vi "Calculate Feedforward.vi"() -> ()   [LabVIEW 2015]
uses:
  <vilib>/Rock Robotics/WPI/CAN/TalonSRX/WPI_CANTalonSRX_APIControlMode.ctl
  <vilib>/Rock Robotics/WPI/MotorControl/WPI_MotorControlOpenCANTalonSRX.vi
panel:
  out "Deltas":dbl[](array[numeric])
  out "Sensor Velocity":dbl[](array[numeric])
  out "Motor Setpoints":dbl[](array[numeric])
  out "Feedfoward(s)":dbl[](array[numeric])
  in  "Motor Inverts":bool[](array[boolean])
  in  "Motor IDs":u8[][](array[numeric])
  out "Valid Data":bool
  out "Velocity Chart (in array order)":cluster{"[0]":dbl, "[1]":dbl}(graph)
  in  "Target Output (vbus)":dbl=0.5 format="%#_13g"
  in  "Counts per rev of encoder":i32=1024
  in  "stop":bool
  in  "Start":bool
  in  "size of averaging array":i32
  in  "Valid Delta":dbl format="%#_13g"
  # "The first of every row is the master motor and every motor after that is the slave to thr"
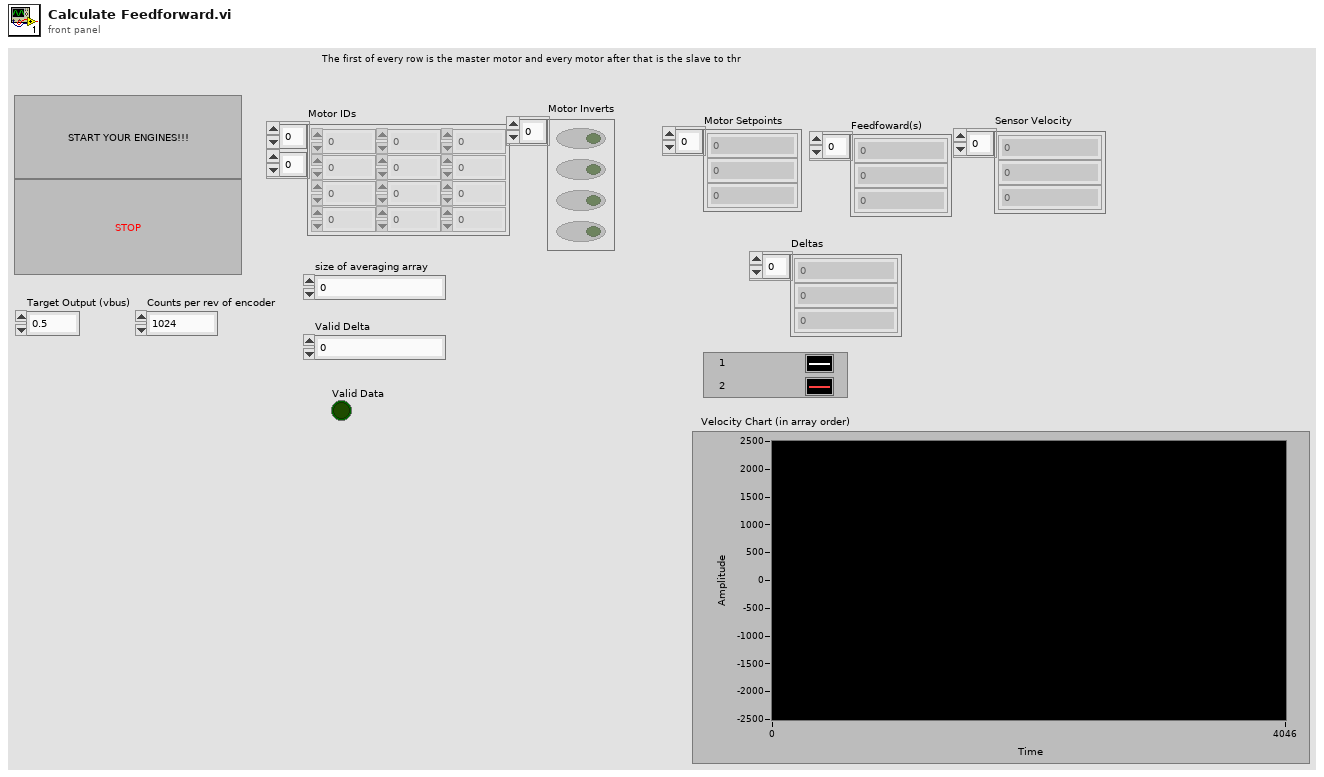
[diagram p1: front panel]
types:
  T1 = typedef "WPI_CANTalonSRX_APIControlMode.ctl" = enum8{"Percent VBus", "Speed", "Position", "Slave", "Unchanged / Invalid", "Voltage Compensation", "Current", "Motion Profile"}
  T2 = typedef "WPI_MotorControlDeviceRef.ctl" = cluster{"DeviceStatus":errorcluster, "Type":T3, "PWM":cluster{"PWM Channel":T4, "DeadBand":T5}, "CAN":cluster{"Device Number":u8, "Control Mode":T6, "Semaphore":T7, "Max Vout":dbl, "TalonSRX Control Mode":T1}, "Invert":bool}
  T3 = typedef "WPI_MotorControlType.ctl" = enum16{"PWM", "CAN", "CANTalonSRX"}
  T4 = typedef "FPGA_DIOPWMChannel.ctl" = enum8{"PWM 0", "PWM 1", "PWM 2", "PWM 3", "PWM 4", "PWM 5", "PWM 6", "PWM 7", "PWM 8", "PWM 9", "PWM MXP 0", "PWM MXP 1", "PWM MXP 2", "PWM MXP 3", "PWM MXP 4", "PWM MXP 5", "PWM MXP 6", "PWM MXP 7", "PWM MXP 8", "PWM MXP 9", "Invalid"}
  T5 = typedef "WPI_PWMDeadband.ctl" = cluster{"Name":string, "maxPositivePwm":i32, "minPositivePwm":i32, "centerPwm":i32, "maxNegativePwm":i32, "minNegativePwm":i32, "angularRange":u16}
  T6 = typedef "WPI_CANJaguar_ControlMode.ctl" = enum8{"Percent VBus", "Current", "Speed", "Position", "Voltage"}
  T7 = typedef "Semaphore RefNum" = refnum<k1>
  T8 = typedef "WPI_CANTalonSRX_GlobalStatus.ctl" = cluster{"Applied Throttle":dbl, "Module Enabled":bool, "CAN Error":errorcluster, "Closed Loop Error":dbl, "Forward Limit Switch Closed":bool, "Reverse Limit Switch Closed":bool, "Sensor Position":dbl, "Sensor Velocity":dbl, "Current":dbl, "Sticky Fault - Over Temp":bool, "Sticky Fault - Under Voltage":bool, "Sticky Fault - Forward Limit":bool, "Sticky Fault - Reverse Limit":bool, "Sticky Fault - Forward Soft Limit":bool, "Sticky Fault - Reverse Soft Limit":bool, "Brake is Enabled":bool, "Encoder Position":dbl, "Encoder Velocity":dbl, "Encoder Index Count":dbl, "Encoder A Pin State":bool, "Encoder B Pin State":bool, "Encoder Index Pin State":bool, "Analog In":dbl, "Analog In Velocity":dbl, "Temperature (C)":dbl, "Battery Voltage":dbl, "Control 5 Is Supported":bool, "Current Profile Slot Select":dbl, "Pos Div 8":bool, "Vel Div 4":bool, "Pulse Width Position":i32, "Pulse Width Velocity":i32, "Pulse Width Rise To Rise (us)":i32, "Pulse Width Rise To Fall (us)":i32, "Mot Prof Active Is Under Run":bool, "Mot Prof Active Has Under Run":bool, "Mot Prof Active Is Last":bool, "Mot Prof Active Velocity Only":bool, "Mot Prof Active Is Valid":bool, "Mot Prof Buffer Is Full":bool, "Mot Prof Active Profile Slot Select":i32, "Mot Prof NextID":i32, "Mot Prof Count":i32, "Mot Prof Active Velocity":dbl, "Mot Prof Active Position":dbl, "Mot Prof Output Enable":i32}
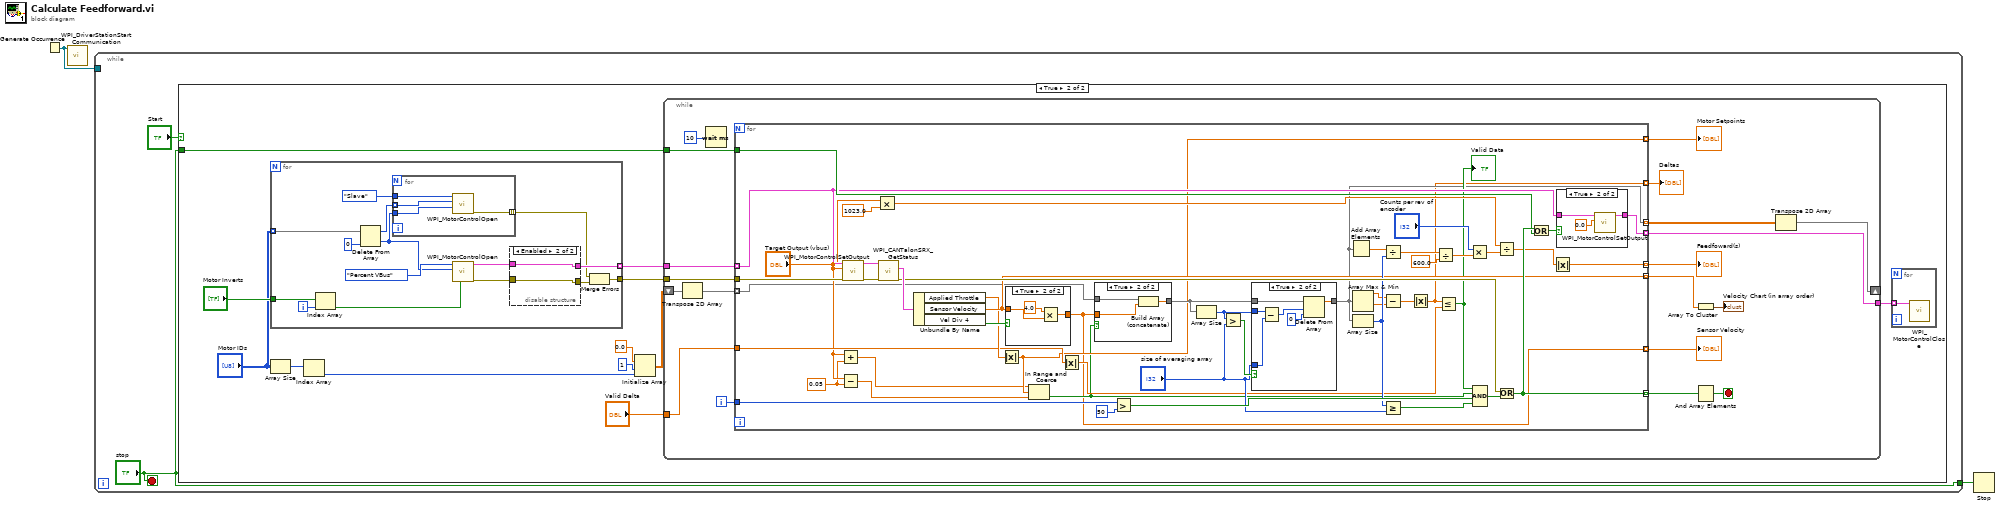
[diagram p0: block diagram]
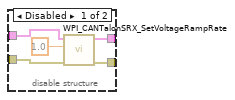
[diagram p3: hidden frame]
diagram:
  n1 = Generate Occurrence() -> (w2:refnum<k4>)
  n2 = call <vilib>:"WPI_DriverStationStart Communication.vi"("occurrence"=w2) -> ()  [unwired: 1 in, 10 out]
  n3 = while {
    tunnel: w2 -> [_]
    tunnel: ["stop"] -> w1
    stop <- "stop" stop-if-true
    n4 = case shown="True" "Start" {
      tunnel: "stop" -> [_ w13]
      frame False {
      }
      frame True {
        n5 = for {
          tunnel: [w27] -> w14
          tunnel: "Motor IDs" -> [w26] mode=indexing
          tunnel: [w29] -> w12 mode=indexing
          tunnel: "Motor Inverts" -> [w18]
          i -> [w20]
          n6 = Index Array(array=w18, index=w20) -> (element=w19:bool)
          n7 = Delete From Array(array=w26, index=0) -> (deleted portion=w23:u8, array with subset deleted=w24:u8[])  [unwired: 1 in]
          n8 = for {
            tunnel: w24 -> [w43] mode=indexing
            tunnel: w23 -> [w42]
            tunnel: WPI_CANTalonSRX_APIControlMode."Slave" ("Control Mode") -> [w41]
            tunnel: [w40] -> w21 mode=indexing
            n9 = call-poly <vilib>:"WPI_MotorControlOpen.vi"("Master Device Number"=w42, "Device Number"=w43, "Control Mode"=w41) -> ("error out"=w40:errorcluster)  [unwired: 7 in, 1 out]
          }
          n10 = call-poly <vilib>:"WPI_MotorControlOpen.vi"("Invert"=w19, "Device Number"=w23, "Control Mode"=WPI_CANTalonSRX_APIControlMode."Percent VBus") -> ("error out"=w30:errorcluster, "MotorControlDeviceRef"=w31:T2)  [unwired: 7 in]
          n11 = disable-structure shown="Enabled" {
            disable-tunnel: w31 -> [w36 w39]
            disable-tunnel: w30 -> [w35 w38]
            disable-tunnel: [w34 w39] -> w29
            disable-tunnel: [w33 w38] -> w28
            frame Disabled {
              n12 = call <vilib>:"WPI_CANTalonSRX_SetVoltageRampRate.vi"("error in (no error)"=w35, "Throttle Ramp Rate (percent/s)"=1.0, "CAN Talon SRX Ref"=w36) -> ("error out"=w33:errorcluster, "CAN Talon SRX Ref"=w34:T2)  [unwired: 7 in]
            }
            frame Enabled {
            }
          }
          n13 = Merge Errors(w21, w28) -> (w27:errorcluster)
        }
        n14 = Array Size(array="Motor IDs") -> (size(s)=w8:i32[])
        n15 = Index Array(array=w8) -> (element=w6:i32)  [unwired: 1 in]
        n16 = Initialize Array(0.0 ("element"), 1 ("dimension size"), w6) -> (w7:dbl[][])
        n17 = while {
          tunnel: w12 -> [w56]
          tunnel: "Valid Delta" -> [w62]
          shift-right: [w47] -> _
          shift-left: w7 -> [w49]
          tunnel: [w55] -> w15
          tunnel: w14 -> [w59]
          tunnel: w13 -> [w57]
          i -> [w60]
          stop <- w44 stop-if-true
          n18 = Transpose 2D Array(2D array=w49) -> (transposed array=w48:dbl[][])
          n19 = Wait (ms)(milliseconds to wait=u32 10) -> ()  [unwired: 1 out]
          n20 = for {
            tunnel: w62 -> [w75]
            tunnel: w48 -> [w66] mode=indexing
            tunnel: w60 -> [w105]
            tunnel: w59 -> [w101]
            tunnel: [w93] -> w58 mode=indexing
            tunnel: w57 -> [w92]
            tunnel: w56 -> [w84] mode=indexing
            tunnel: [w83] -> w55 mode=indexing
            tunnel: [w65] -> w54 mode=indexing
            tunnel: [w81] -> w53 mode=indexing
            tunnel: [w73] -> w51 mode=indexing
            tunnel: [w67] -> w50 mode=indexing
            tunnel: [w64] -> w46 mode=indexing
            tunnel: [w63] -> w45 mode=indexing
            w70 = 0.05 ("y")
            n21 = Add(x="Target Output (vbus)", y=w70) -> (x+y=w72:dbl)
            n22 = Subtract(x="Target Output (vbus)", y=w70) -> (x-y=w69:dbl)
            n23 = call <vilib>:"WPI_MotorControlSetOutput.vi"("error in (no error)"=w101, "Output"="Target Output (vbus)", "MotorControlDevRef"=w84) -> ("error out"=w100:errorcluster, "MotorControlDevRef"=w106:T2)  [unwired: 6 in, 1 out]
            n24 = Multiply(x="Target Output (vbus)", y=1023.0 ("x")) -> (x*y=w85:dbl)
            n25 = call <vilib>:"WPI_CANTalonSRX_GetStatus.vi"("error in (no error)"=w100, "CAN Talon SRX Ref"=w106) -> ("error out"=w99:errorcluster, "Talon SRX Status"=w111:T8)  [unwired: 7 in, 1 out]
            n26 = Unbundle By Name(w111) -> ("Applied Throttle"=w80:dbl, "Sensor Velocity"=w81:dbl, "Vel Div 4"=w94:bool)
            n27 = Absolute Value(x=w80) -> (abs(x)=w73:dbl)
            n28 = case shown="True" w94 {
              tunnel: [w112 w113] -> w64
              tunnel: w81 -> [w112 w114]
              frame False {
              }
              frame True {
                n29 = Multiply(x=4.0, y=w114) -> (x*y=w113:dbl)
              }
            }
            n30 = In Range and Coerce(upper limit=w72, x=w73, lower limit=w69) -> (In Range?=w68:bool)  [unwired: 1 out]
            n31 = Absolute Value(x=w75) -> (abs(x)=w76:dbl)
            n32 = case shown="True" w68 {
              tunnel: w66 -> [w116 w119]
              tunnel: [w116 w118] -> w109
              tunnel: w64 -> [_ w117]
              frame False {
              }
              frame True {
                n33 = Build Array (concatenate)(w119, w117) -> (w118:dbl[])
              }
            }
            n34 = Greater?(x=w105, y=50) -> (0:w103:bool)
            n35 = Array Size(array=w109) -> (size(s)=w108:i32)
            n36 = Greater?(x=w108, y="size of averaging array") -> (0:w110:bool)
            n37 = case shown="True" w110 {
              tunnel: w109 -> [w124 w130]
              tunnel: "size of averaging array" -> [_ w129]
              tunnel: w108 -> [_ w128]
              tunnel: [w124 w125] -> w67
              frame False {
              }
              frame True {
                n38 = Subtract(x=w128, y=w129) -> (x-y=w127:i32)
                n39 = Delete From Array(array=w130, length=w127, index=0) -> (array with subset deleted=w125:dbl[])  [unwired: 1 out]
              }
            }
            n40 = Add Array Elements(numeric array=w67) -> (sum=w107:dbl)
            n41 = Array Max & Min(array=w67) -> (max value=w79:dbl, min value=w78:dbl)  [unwired: 2 out]
            n42 = Array Size(array=w67) -> (size(s)=w97:i32)
            n43 = Divide(x=w107, y=w97) -> (x/y=w90:dbl)
            n44 = Subtract(x=w79, y=w78) -> (x-y=w77:dbl)
            n45 = Greater Or Equal?(x=w97, y="size of averaging array") -> (x >= y?=w95:bool)
            n46 = Absolute Value(x=w77) -> (abs(x)=w63:dbl)
            n47 = Divide(x=w90, y=600.0) -> (x/y=w87:dbl)
            n48 = Less Or Equal?(x=w63, y=w76) -> (x <= y?=w74:bool)
            "Valid Data" <- w74
            n49 = Multiply(x="Counts per rev of encoder", y=w87) -> (x*y=w86:dbl)
            n50 = Compound Arithmetic op=AND(w74, w68, w103, w95) -> (w102:bool)
            n51 = Divide(x=w85, y=w86) -> (x/y=w82:dbl)
            n52 = Or(x=w99, y=w102) -> (x .or. y?=w93:bool)
            n53 = Or(x=w93, y=w92) -> (x .or. y?=w91:bool)
            n54 = Absolute Value(x=w82) -> (abs(x)=w65:dbl)
            n55 = case shown="True" w91 {
              tunnel: w84 -> [w120 w122]
              tunnel: [w120 w121] -> w83
              frame False {
              }
              frame True {
                n56 = call <vilib>:"WPI_MotorControlSetOutput.vi"("Output"=0.0, "MotorControlDevRef"=w122) -> ("MotorControlDevRef"=w121:T2)  [unwired: 7 in, 2 out]
              }
            }
          }
          "Feedfoward(s)" <- w54
          "Motor Setpoints" <- w51
          "Sensor Velocity" <- w46
          "Deltas" <- w45
          n57 = Array To Cluster(array=w53) -> (cluster=→"Velocity Chart (in array order)":cluster{"[0]":dbl, "[1]":dbl})
          n58 = And Array Elements(Boolean array=w58) -> (logical AND=w44:bool)
          n59 = Transpose 2D Array(2D array=w50) -> (transposed array=w47:dbl[][])
        }
        n60 = for {
          tunnel: w15 -> [w17] mode=indexing
          n61 = call <vilib>:"WPI_MotorControlClose.vi"("MotorControlDevRef"=w17) -> ()  [unwired: 10 in, 1 out]
        }
      }
    }
  }
  n62 = Stop(stop? (T)=w1) -> ()
